vi "Do.vi"(8 "error in (no error)":errorcluster, 10 "Actor in":refnum<class "Actor.lvclass">, 11 "Update_buy_values Msg":refnum<class "Update_buy_values Msg.lvclass">) -> (0 "error out":errorcluster, 2 "Actor out":refnum<class "Actor.lvclass">)   [LabVIEW 2019, in "UI Actor.lvlib" / "Update_buy_values Msg.lvclass"]
doc: "This VI delivers the message to the actor by calling the appropriate method(s) on the actor."
uses:
  Update_buy_values Msg.lvclass
  <vilib>/ActorFramework/Actor/Actor.lvclass
  UI Actor/UI Actor.lvclass
  C:/Program Files/National Instruments/LabVIEW 2019/vi.lib/ActorFramework/Actor/Actor.lvclass
  Update_buy_values Msg.lvclass/Update_buy_values Msg.ctl
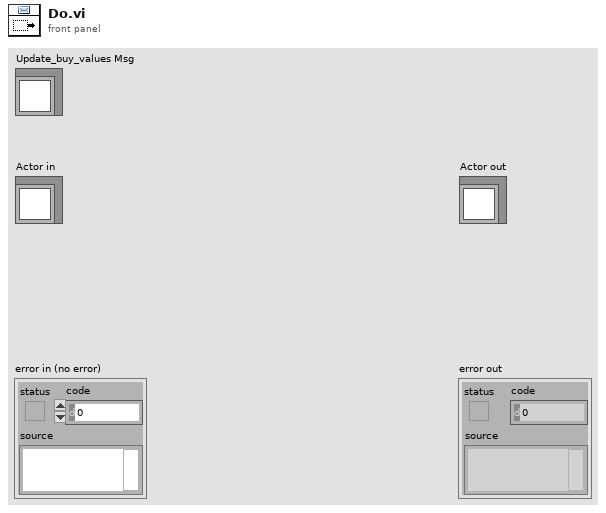
[diagram p1: front panel]
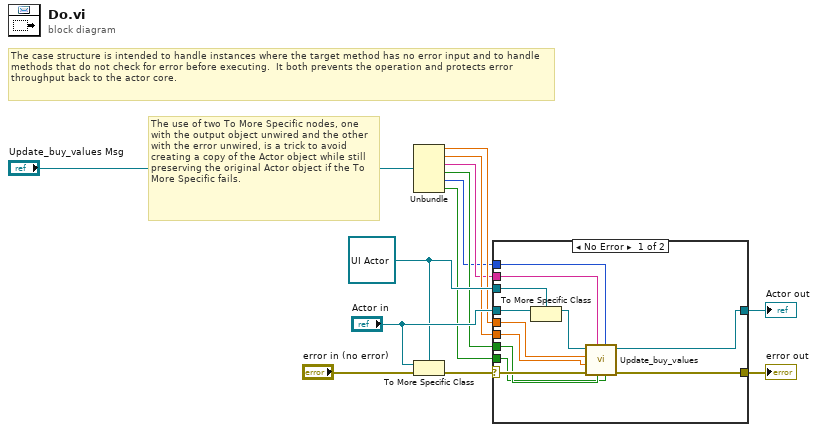
[diagram p0: block diagram]
diagram:
  w8 = refnum<class "UI Actor.lvclass"> refnum ("Actor in")
  # "The use of two To More Specific nodes, one with the output object unwired and the other with the error unwired, is a trick to avoid creating a copy of the Actor object while still preserving the original Actor object if the To More Specific fails."
  # "The case structure is intended to handle instances where the target method has no error input and to handle methods that do not check for error before executing.  It both prevents the operation and protects error throughput back to the actor core."
  n1 = Unbundle("Update_buy_values Msg") -> (w6:dbl, w5:dbl, w4:string, w3:bool, w2:i32, w1:bool)
  n2 = To More Specific Class(target class=w8, reference="Actor in", error in="error in (no error)") -> (error out=w7:errorcluster)  [unwired: 1 out]
  n3 = case shown="No Error" w7 {
    selector: w7 -> [w23 w27]
    tunnel: [w25 w27] -> w13
    tunnel: [w24 w26] -> w12
    tunnel: "Actor in" -> [w22 w26]
    tunnel: w8 -> [w21 _]
    tunnel: w6 -> [w19 _]
    tunnel: w5 -> [w18 _]
    tunnel: w4 -> [w17 _]
    tunnel: w3 -> [w16 _]
    tunnel: w2 -> [w15 _]
    tunnel: w1 -> [w14 _]
    frame No Error {
      n4 = To More Specific Class(target class=w21, reference=w22) -> (specific class reference=w20:refnum<class "UI Actor.lvclass">)  [unwired: 1 in, 1 out]
      n5 = call "Update_buy_values.vi"("SODA?"=w14, "Index"=w15, "MXN?"=w16, "Producto"=w17, "error in (no error)"=w23, "Cantidad"=w18, "Precio"=w19, "UI Actor in"=w20) -> ("error out"=w25:errorcluster, "UI Actor out"=w24:refnum<class "UI Actor.lvclass">)  [unwired: 2 in]
    }
    frame Error {
      # "If type check fails, pass the original object out again."
    }
  }
  "error out" <- w13
  "Actor out" <- w12
